vi "PH_ImageCalibrator.get Text for Save Result Dialog.vi"(0 "i ref in":refnum<vi>, 5 "error in (no error)":errorcluster) -> (14 "i ref out":refnum<vi>, 17 "User Dialog":string, 19 "error out":errorcluster)   [LabVIEW 2014, in "PH_ImageCalibrator.lvlib"]
doc: "Thi VI checks whether all data are taken with sucess to set the User Dialog."
uses:
  PH_ImageCalibrator.lvlib
  PH_Basics/PH_Img_BaseClass/PH_Img_BaseClass.lvlib
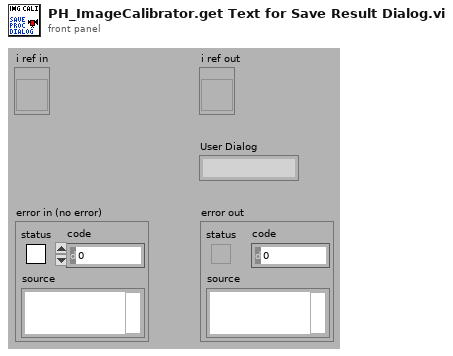
[diagram p1: front panel]
types:
  T1 = typedef "PH_ImageCalibrator.lvlib/PH_ImageCalibrator.i attribute.ctl" = cluster{"GUI Refs":cluster{"Available Cams":refnum<vi>, "OK":refnum<vi>, "Skip":refnum<vi>, "Repeat":refnum<vi>, "Cancel":refnum<vi>, "Length [mm]":refnum<vi>, "Energy [mJ]":refnum<vi>, "Dialog":refnum<vi>}, "Cam instances":string[], "Dark Pics":cluster{"#":i32, "BI taken":bool}, "Lin Cali":cluster{"Distance [Pixel]":dbl, "Distance [mm]":dbl, "Lin Cali Factor [mm/Pixel]":dbl}, "Energy Cali":cluster{"Pixelsum":dbl, "Energy [mJ]":dbl, "Energy Cali factor [mJ/Pixelsum]":dbl, "Underground subtracted?":bool, "#":i32}, "Images":cluster{"Background":T2, "Energy":T2}}
  T2 = typedef "IMAQ Image.ctl" = refnum<image>
  T3 = typedef "PH_Img_BaseClass.lvlib/PH_Img_BaseClass.i attribute.ctl" = cluster{"GUI Refs":T4, "Timeout Image [ms]":i32, "Default Periodic Period [ms]":i32, "Camera":cluster{"Instancename":string, "Notifier":refnum<notifier>}, "Palette":T5, "Cam Settings":cluster{"Cam ID":string, "Gain":dbl, "Brightness":dbl, "Shutter":dbl, "Cam Info Failure":bool, "Mode":i32}}
  T4 = typedef "PH_Img_BaseClass.lvlib/PH_Img_BaseClass.GUI Refs.ctl" = cluster{"Timeout":refnum<vi>, "Image":refnum<vi>, "Palette":refnum<vi>, "Timeout Set":refnum<vi>}
  T5 = typedef "PH_Img_BaseClass.lvlib/PH_Img_BaseClass.Palette.ctl" = i32
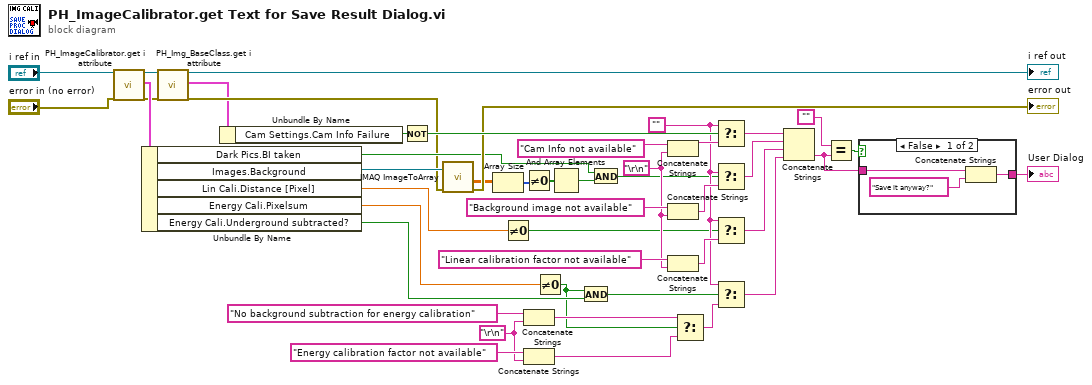
[diagram p0: block diagram]
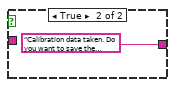
[diagram p2: hidden frame]
diagram:
  w25 = "\r\n"
  w31 = ""
  w24 = "\r\n"
  n1 = call "PH_ImageCalibrator.get i attribute.vi"("i ref in"="i ref in", "error in (no error)"="error in (no error)") -> ("i ref out"=w4:refnum<vi>, "i attribute"=w44:T1, "error out"=w12:errorcluster)  [unwired: 15 in]
  n2 = Unbundle By Name(w44) -> ("Dark Pics.BI taken"=w7:bool, "Images.Background"=w6:T2, "Lin Cali.Distance [Pixel]"=w34:dbl, "Energy Cali.Pixelsum"=w33:dbl, "Energy Cali.Underground subtracted?"=w20:bool)
  n3 = call "PH_Img_BaseClass.get i attribute.vi"("i ref in"=w4, "error in (no error)"=w12) -> ("i ref out"=→"i ref out":refnum<vi>, "i attribute"=w2:T3, "error out"=w5:errorcluster)  [unwired: 15 in]
  n4 = Unbundle By Name(w2) -> ("Cam Settings.Cam Info Failure"=w1:bool)
  n5 = Not(x=w1) -> (.not. x?=w41:bool)
  n6 = call "IMAQ ImageToArray"("error in (no error)"=w5, "Image"=w6) -> ("Image Pixels (Float)"=w10:sgl[][], "error out"=→"error out":errorcluster)  [unwired: 2 in, 3 out]
  n7 = Array Size(array=w10) -> (size(s)=w43:i32[])
  n8 = Not Equal To 0?(x=w34) -> (x != 0?=w21:bool)
  n9 = Not Equal To 0?(x=w43) -> (x != 0?=w42:bool[])
  n10 = Concatenate Strings("No background subtraction for energy calibration", w25) -> (w26:string)
  n11 = Concatenate Strings("Energy calibration factor not available", w25) -> (w28:string)
  n12 = Not Equal To 0?(x=w33) -> (x != 0?=w19:bool)
  n13 = And Array Elements(Boolean array=w42) -> (logical AND=w9:bool)
  n14 = And(x=w19, y=w20) -> (x .and. y?=w32:bool)
  n15 = And(x=w7, y=w9) -> (x .and. y?=w8:bool)
  n16 = Concatenate Strings("Cam Info not available", w24) -> (w39:string)
  n17 = Concatenate Strings("Background image not available", w24) -> (w38:string)
  n18 = Concatenate Strings("Linear calibration factor not available", w24) -> (w35:string)
  n19 = Select(t=w26, s=w19, f=w28) -> (s? t:f=w30:string)
  n20 = Select(t=w31, s=w41, f=w39) -> (s? t:f=w23:string)
  n21 = Select(t=w31, s=w8, f=w38) -> (s? t:f=w22:string)
  n22 = Select(t=w31, s=w21, f=w35) -> (s? t:f=w18:string)
  n23 = Select(t=w31, s=w32, f=w30) -> (s? t:f=w17:string)
  n24 = Concatenate Strings(w23, w22, w18, w17) -> (w13:string)
  n25 = Equal?(x="" ("y"), y=w13) -> (x = y?=w16:bool)
  n26 = case shown="False" w16 {
    tunnel: [w49 "Calibration data taken. Do you want to save the result?"] -> w14
    tunnel: w13 -> [w47 _]
    frame False {
      n27 = Concatenate Strings(w47, "Save it anyway?") -> (w49:string)
    }
    frame True {
    }
  }
  "User Dialog" <- w14
